vi "SetSide.vi"(8 "error in (no error)":errorcluster, 9 "MapSite*":refnum<data-value>, 10 "Direction":T1, 11 "Room in":refnum<class "Room.lvclass">) -> (0 "error out":errorcluster, 3 "Room out":refnum<class "Room.lvclass">)   [LabVIEW 2016, in "Room.lvclass"]
uses:
  Room.lvclass
  Direction.ctl
  MapSite/MapSite.lvclass
  Room.lvclass/Room.ctl
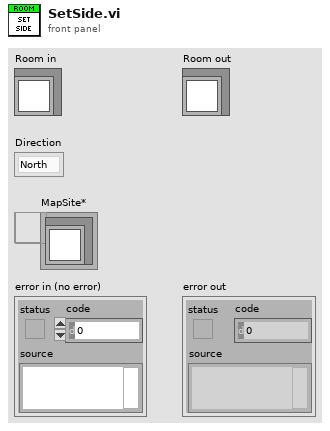
[diagram p1: front panel]
types:
  T1 = typedef "Room.lvclass/Direction.ctl" = enum16{"North", "South", "East", "West"}
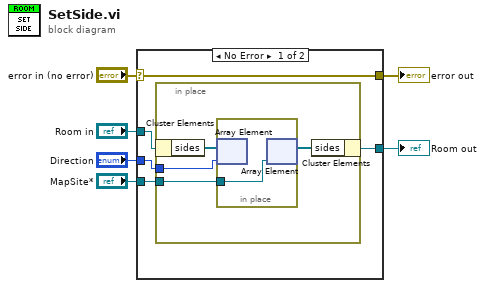
[diagram p0: block diagram]
diagram:
  n1 = case shown="No Error" "error in (no error)" {
    selector: "error in (no error)" -> [w11 w18]
    tunnel: [w11 w18] -> w5
    tunnel: [w7 w17] -> w3
    tunnel: "Room in" -> [w10 w17]
    tunnel: "Direction" -> [w9 _]
    tunnel: "MapSite*" -> [w8 _]
    frame No Error {
      n2 = in-place {
        in-place-border: w9 -> [w14]
        in-place-border: w8 -> [w13]
        n3 = in-place-cluster #1(w10) -> ("sides"=w15:refnum<data-value>[])
        n4 = in-place {
          in-place-border: w13 -> [w16]
          n5 = in-place-array #2(w15, w14) -> ()  [unwired: 1 out]
          n6 = in-place-array #2(w16) -> (w12:refnum<data-value>[])  [unwired: 1 out]
        }
        n7 = in-place-cluster #1("sides"=w12) -> (w7:refnum<class "Room.lvclass">)
      }
    }
    frame Error {
    }
  }
  "error out" <- w5
  "Room out" <- w3
